vi "To Integer Tree Data.vi"(10 "Integer":i64) -> (3 "Integer Tree Data":refnum<class "Integer.lvclass">)   [LabVIEW 2016, in "Integer.lvclass"]
uses:
  Integer.lvclass
  Integer.lvclass/Integer.ctl
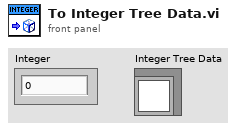
[diagram p1: front panel]
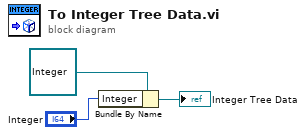
[diagram p0: block diagram]
diagram:
  n1 = Bundle By Name(cluster=refnum<class "Integer.lvclass"> refnum ("Int in"), "Integer"="Integer") -> (→"Integer Tree Data":refnum<class "Integer.lvclass">)
